vi "myRIO_BRig_RT_dataExp_laser2_Freq.vi"() -> (2 "output_laser2_Freq":i32)   [LabVIEW 2014]
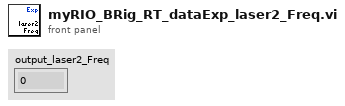
[diagram p1: front panel]
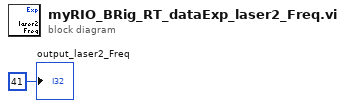
[diagram p0: block diagram]
diagram:
  "output_laser2_Freq" <- 41 ("output_iBlock")
